vi "Obtain Request Events.vi"(8 "error in (no error)":errorcluster, 10 "Create New?":bool) -> (0 "error out":errorcluster, 2 "UI Manager Request Events":T1)   [LabVIEW 2022 SP3, in "UI Manager.lvlib"]
doc: "This VI Obtains/Creates the Requests events that will be used for other modules to communicate with the module that owns this VI. These Requests events will be accessed only via Public API methods for this module.\n\n<b>NOTE</b>: The contents of this VI are automatically generated and modified by the <b>Tools > Delacor > DQMH</b> utilities. Consider using those utilities instead of making your own modifications to this VI.\n____\nHAMPEL SOFTWARE ENGINEERING v2.6.0 (2023-12-19 10:54)"
uses:
  UI Manager.lvlib
  Request Events--cluster.ctl
  Stop Argument--cluster.ctl
  Show Panel Argument--cluster.ctl
  Hide Panel Argument--cluster.ctl
  Get Module Execution Status Argument--cluster.ctl
  Show Diagram Argument--cluster.ctl
  Set Run-Time Menu Argument--cluster.ctl
  Show HSE-ABOUT Argument--cluster.ctl
  Show PROJECT-ABOUT Argument--cluster.ctl
  Configure Argument--cluster.ctl
  Prepare Argument--cluster.ctl
  Update Status Bar Argument--cluster.ctl
  Trigger System Message Argument--cluster.ctl
  Add Module to Run-Time Menu Argument--cluster.ctl
  Set Modules Argument--cluster.ctl
  Set Modules (Reply Payload)--cluster.ctl
  Register for Module Events Argument--cluster.ctl
  Libraries/hse-libraries/Source/hse-dqmh/Controls/System Message Argument--cluster.ctl
  Libraries/hse-libraries/Source/hse-dqmh/Controls/System Message Source.ctl
  Display another Module UI Argument--cluster.ctl
  Module Display Scenarios.ctl
  Set Run-Time Menu Visibility Argument--cluster.ctl
  Set Window Closeable State Argument--cluster.ctl
  Shutdown Application Argument--cluster.ctl
  Remove Module from Run-Time Menu Argument--cluster.ctl
  Set CLI Arguments Argument--cluster.ctl
  Set CLI Arguments (Reply Payload)--cluster.ctl
  Get CLI Arguments Argument--cluster.ctl
  Get CLI Arguments (Reply Payload)--cluster.ctl
  External Login Argument--cluster.ctl
  Get User Level Argument--cluster.ctl
  Get User Level (Reply Payload)--cluster.ctl
  Libraries/hse-libraries/Source/hse-dqmh/hse-dqmh.lvlib
panel:
  # "NOTE: The contents of this VI are automatically generated and modified by the Tools > Delacor > DQMH utilities. Consider using those utilities instead of making your own modifications to this VI."
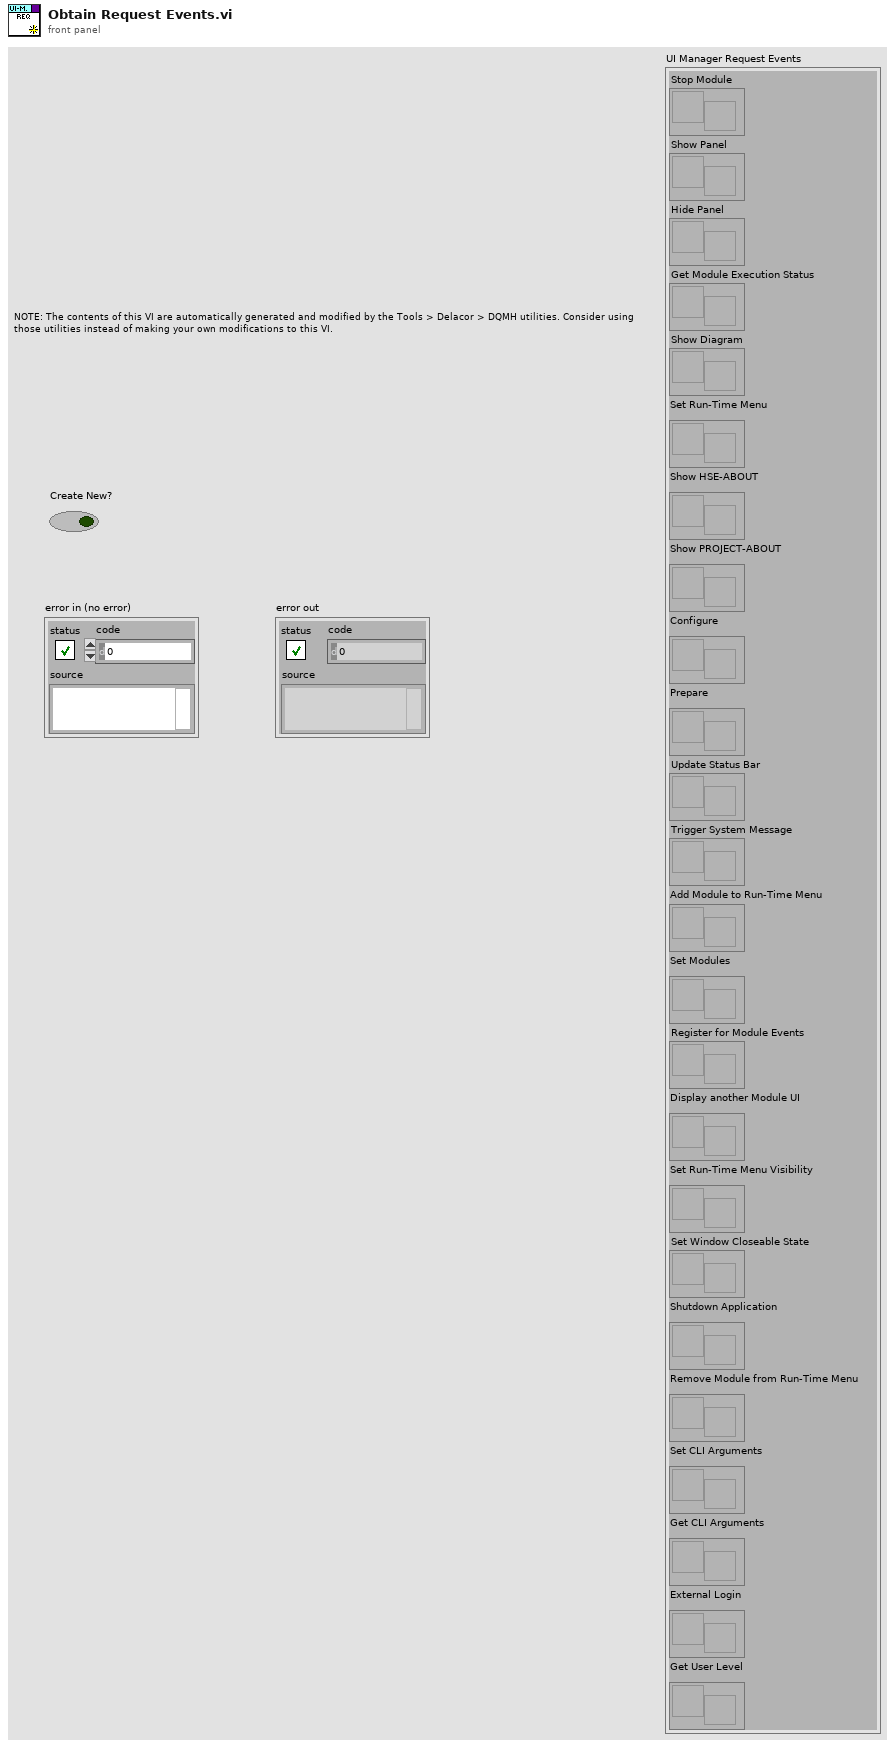
[diagram p1: front panel]
types:
  T1 = typedef "UI Manager.lvlib/Request Events--cluster.ctl" = cluster{"Stop Module":refnum<user-event>, "Show Panel":refnum<user-event>, "Hide Panel":refnum<user-event>, "Get Module Execution Status":refnum<user-event>, "Show Diagram":refnum<user-event>, "Set Run-Time Menu":refnum<user-event>, "Show HSE-ABOUT":refnum<user-event>, "Show PROJECT-ABOUT":refnum<user-event>, "Configure":refnum<user-event>, "Prepare":refnum<user-event>, "Update Status Bar":refnum<user-event>, "Trigger System Message":refnum<user-event>, "Add Module to Run-Time Menu":refnum<user-event>, "Set Modules":refnum<user-event>, "Register for Module Events":refnum<user-event>, "Display another Module UI":refnum<user-event>, "Set Run-Time Menu Visibility":refnum<user-event>, "Set Window Closeable State":refnum<user-event>, "Shutdown Application":refnum<user-event>, "Remove Module from Run-Time Menu":refnum<user-event>, "Set CLI Arguments":refnum<user-event>, "Get CLI Arguments":refnum<user-event>, "External Login":refnum<user-event>, "Get User Level":refnum<user-event>}
  T2 = typedef "UI Manager.lvlib/Get User Level Argument--cluster.ctl" = cluster{"Wait Notifier":refnum<notifier>, "wait for reply":bool}
  T3 = typedef "UI Manager.lvlib/External Login Argument--cluster.ctl" = cluster{"User Name":string, "User Level":string}
  T4 = typedef "UI Manager.lvlib/Get CLI Arguments Argument--cluster.ctl" = cluster{"Wait Notifier":refnum<notifier>, "wait for reply":bool}
  T5 = typedef "UI Manager.lvlib/Set CLI Arguments Argument--cluster.ctl" = cluster{"CLI Arguments":string[], "Wait Notifier":refnum<notifier>, "wait for reply":bool}
  T6 = typedef "UI Manager.lvlib/Remove Module from Run-Time Menu Argument--cluster.ctl" = cluster{"Module DQMH Path":path}
  T7 = typedef "UI Manager.lvlib/Shutdown Application Argument--cluster.ctl" = cluster{"User Confirm?":bool}
  T8 = typedef "UI Manager.lvlib/Set Window Closeable State Argument--cluster.ctl" = cluster{"Closeable?":bool}
  T9 = typedef "UI Manager.lvlib/Set Run-Time Menu Visibility Argument--cluster.ctl" = cluster{"Visible?":bool}
  T10 = typedef "UI Manager.lvlib/Display another Module UI Argument--cluster.ctl" = cluster{"Module DQMH Path":path, "Display Scenario":T11}
  T11 = typedef "UI Manager.lvlib/Module Display Scenarios.ctl" = enum16{"Stand-Alone", "Managed"}
  T12 = typedef "UI Manager.lvlib/Register for Module Events Argument--cluster.ctl" = cluster{"System Messages":refnum<user-event>[]}
  T13 = typedef "UI Manager.lvlib/Set Modules Argument--cluster.ctl" = cluster{"Module Paths":path[], "Wait Notifier":refnum<notifier>, "wait for reply":bool}
  T14 = typedef "UI Manager.lvlib/Add Module to Run-Time Menu Argument--cluster.ctl" = cluster{"Module DQMH Path":path, "Module Descriptor":string}
  T15 = typedef "UI Manager.lvlib/Trigger System Message Argument--cluster.ctl" = cluster{"Boolean":bool}
  T16 = typedef "UI Manager.lvlib/Update Status Bar Argument--cluster.ctl" = cluster{"Status Message":string}
  T17 = typedef "UI Manager.lvlib/Prepare Argument--cluster.ctl" = cluster{"Boolean":bool}
  T18 = typedef "UI Manager.lvlib/Configure Argument--cluster.ctl" = cluster{"Boolean":bool}
  T19 = typedef "UI Manager.lvlib/Show PROJECT-ABOUT Argument--cluster.ctl" = cluster{"Boolean":bool}
  T20 = typedef "UI Manager.lvlib/Show HSE-ABOUT Argument--cluster.ctl" = cluster{"Boolean":bool}
  T21 = typedef "UI Manager.lvlib/Set Run-Time Menu Argument--cluster.ctl" = cluster{"Run-Time Menu Path":path}
  T22 = typedef "UI Manager.lvlib/Hide Panel Argument--cluster.ctl" = cluster{"Hide Panel?":bool}
  T23 = typedef "UI Manager.lvlib/Show Panel Argument--cluster.ctl" = cluster{"Show Panel?":bool}
  T24 = typedef "UI Manager.lvlib/Show Diagram Argument--cluster.ctl" = cluster{"Debug?":bool}
  T25 = typedef "UI Manager.lvlib/Get Module Execution Status Argument--cluster.ctl" = cluster{"Running?":bool}
  T26 = typedef "UI Manager.lvlib/Stop Argument--cluster.ctl" = cluster{"Origin":string, "Exit via Stop Module Req?":bool, "Wait for Module to stop?":bool}
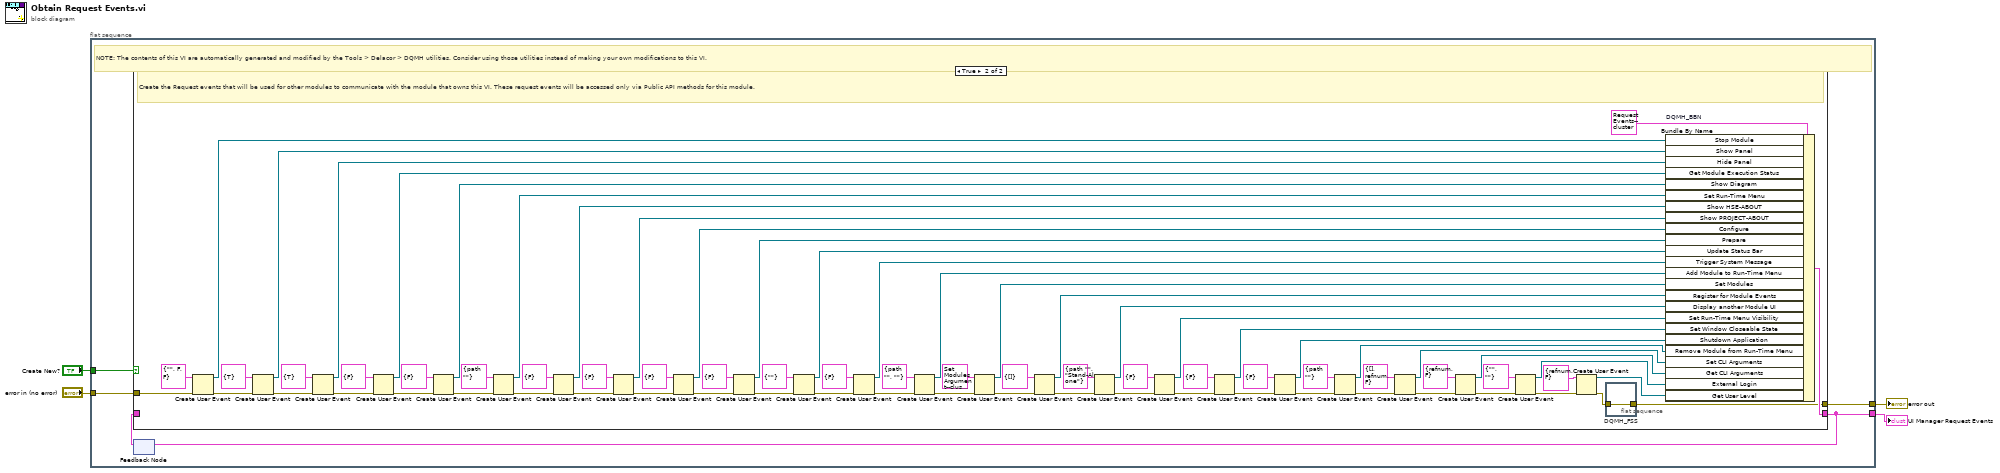
[diagram p0: block diagram]
diagram:
  n1 = flat-sequence {
    tunnel: [w9] -> w4
    tunnel: "error in (no error)" -> [w8]
    tunnel: [w6] -> w2
    tunnel: "Create New?" -> [w5]
    frame #0 {
      # "NOTE: The contents of this VI are automatically generated and modified by the Tools > Delacor > DQMH utilities. Consider using those utilities instead of making your own modifications to this VI."
      n2 = feedback #1() -> (w7:T1)  [unwired: 1 in]
      n3 = case shown="True" w5 {
        tunnel: [w10 w77] -> w9
        tunnel: w8 -> [w10 w87]
        tunnel: [w11 w84] -> w6
        tunnel: w7 -> [w11 _]
        frame False {
          # "Obtain the Request events that were created in a previous call to this VI."
        }
        frame True {
          # "Create the Request events that will be used for other modules to communicate with the module that owns this VI. These request events will be accessed only via Public API methods for this module."
          n4 = Create User Event(user event datatype=T26 {"Origin"="", "Exit via Stop Module Req?"=FALSE, "Wait for Module to stop?"=FALSE} ("Stop Argument"), error in=w87) -> (user event=w85:refnum<user-event>, error out=w82:errorcluster)
          n5 = Create User Event(user event datatype=T23 {"Show Panel?"=TRUE} ("Show Panel Argument"), error in=w82) -> (user event=w81:refnum<user-event>, error out=w80:errorcluster)
          n6 = Create User Event(user event datatype=T22 {"Hide Panel?"=TRUE} ("Hide Panel Argument"), error in=w80) -> (user event=w79:refnum<user-event>, error out=w78:errorcluster)
          n7 = Create User Event(user event datatype=T25 {"Running?"=FALSE} ("Get Module Execution Status Argument"), error in=w78) -> (user event=w75:refnum<user-event>, error out=w76:errorcluster)
          n8 = Create User Event(user event datatype=T24 {"Debug?"=FALSE} ("Show Diagram Argument"), error in=w76) -> (user event=w72:refnum<user-event>, error out=w73:errorcluster)
          n9 = Create User Event(user event datatype=T21 {"Run-Time Menu Path"=path ""} ("Set Run-Time Menu Argument"), error in=w73) -> (user event=w67:refnum<user-event>, error out=w68:errorcluster)
          n10 = Create User Event(user event datatype=T20 {"Boolean"=FALSE} ("Show HSE-ABOUT Argument"), error in=w68) -> (user event=w64:refnum<user-event>, error out=w65:errorcluster)
          n11 = Create User Event(user event datatype=T19 {"Boolean"=FALSE} ("Show PROJECT-ABOUT Argument"), error in=w65) -> (user event=w61:refnum<user-event>, error out=w62:errorcluster)
          n12 = Create User Event(user event datatype=T18 {"Boolean"=FALSE} ("Configure Argument"), error in=w62) -> (user event=w58:refnum<user-event>, error out=w59:errorcluster)
          n13 = Create User Event(user event datatype=T17 {"Boolean"=FALSE} ("Prepare Argument"), error in=w59) -> (user event=w55:refnum<user-event>, error out=w56:errorcluster)
          n14 = Create User Event(user event datatype=T16 {"Status Message"=""} ("Update Status Bar Argument"), error in=w56) -> (user event=w52:refnum<user-event>, error out=w53:errorcluster)
          n15 = Create User Event(user event datatype=T15 {"Boolean"=FALSE} ("Trigger System Message Argument"), error in=w53) -> (user event=w49:refnum<user-event>, error out=w50:errorcluster)
          n16 = Create User Event(user event datatype=T14 {"Module DQMH Path"=path "", "Module Descriptor"=""} ("Add Module to Run-Time Menu Argument"), error in=w50) -> (user event=w46:refnum<user-event>, error out=w47:errorcluster)
          n17 = Create User Event(user event datatype=T13 {"Module Paths"=[path "Modules/Dummie"], "Wait Notifier"=refnum, "wait for reply"=FALSE} ("Set Modules Argument"), error in=w47) -> (user event=w43:refnum<user-event>, error out=w44:errorcluster)
          n18 = Create User Event(user event datatype=T12 {"System Messages"=[]} ("Register for Module Events Argument"), error in=w44) -> (user event=w40:refnum<user-event>, error out=w41:errorcluster)
          n19 = Create User Event(user event datatype=T10 {"Module DQMH Path"=path "", "Display Scenario"=enum."Stand-Alone"} ("Display Module UI Argument"), error in=w41) -> (user event=w37:refnum<user-event>, error out=w38:errorcluster)
          n20 = Create User Event(user event datatype=T9 {"Visible?"=FALSE} ("Set Run-Time Menu Visibility Argument"), error in=w38) -> (user event=w34:refnum<user-event>, error out=w35:errorcluster)
          n21 = Create User Event(user event datatype=T8 {"Closeable?"=FALSE} ("Set Window Closeable State Argument"), error in=w35) -> (user event=w31:refnum<user-event>, error out=w32:errorcluster)
          n22 = Create User Event(user event datatype=T7 {"User Confirm?"=FALSE} ("Shutdown Application Argument"), error in=w32) -> (user event=w28:refnum<user-event>, error out=w29:errorcluster)
          n23 = Create User Event(user event datatype=T6 {"Module DQMH Path"=path ""} ("Remove Module from Run-Time Menu Argument"), error in=w29) -> (user event=w25:refnum<user-event>, error out=w26:errorcluster)
          n24 = Create User Event(user event datatype=T5 {"CLI Arguments"=[], "Wait Notifier"=refnum, "wait for reply"=FALSE} ("Broadcast Arguments Argument"), error in=w26) -> (user event=w22:refnum<user-event>, error out=w23:errorcluster)
          n25 = Create User Event(user event datatype=T4 {"Wait Notifier"=refnum, "wait for reply"=FALSE} ("Get CLI Arguments Argument"), error in=w23) -> (user event=w19:refnum<user-event>, error out=w20:errorcluster)
          n26 = Create User Event(user event datatype=T3 {"User Name"="", "User Level"=""} ("External Login Argument"), error in=w20) -> (user event=w16:refnum<user-event>, error out=w17:errorcluster)
          n27 = Create User Event(user event datatype=T2 {"Wait Notifier"=refnum, "wait for reply"=FALSE} ("Get User Level Argument"), error in=w17) -> (user event=w13:refnum<user-event>, error out=w14:errorcluster)
          n28 = flat-sequence "DQMH_FSS" {
            tunnel: w14 -> [w88]
            tunnel: [w88] -> w77
            frame #0 {
            }
          }
          n29 = Bundle By Name "DQMH_BBN"(cluster=T1 {"Stop Module"=refnum, "Show Panel"=refnum, "Hide Panel"=refnum, "Get Module Execution Status"=refnum, "Show Diagram"=refnum, "Set Run-Time Menu"=refnum, "Show HSE-ABOUT"=refnum, "Show PROJECT-ABOUT"=refnum, "Configure"=refnum, "Prepare"=refnum, "Update Status Bar"=refnum, "Trigger System Message"=refnum, "Add Module to Run-Time Menu"=refnum, "Set Modules"=refnum, "Register for Module Events"=refnum, "Display another Module UI"=refnum, "Set Run-Time Menu Visibility"=refnum, "Set Window Closeable State"=refnum, "Shutdown Application"=refnum, "Remove Module from Run-Time Menu"=refnum, "Set CLI Arguments"=refnum, "Get CLI Arguments"=refnum, "External Login"=refnum, "Get User Level"=refnum} ("output cluster"), "Stop Module"=w85, "Show Panel"=w81, "Hide Panel"=w79, "Get Module Execution Status"=w75, "Show Diagram"=w72, "Set Run-Time Menu"=w67, "Show HSE-ABOUT"=w64, "Show PROJECT-ABOUT"=w61, "Configure"=w58, "Prepare"=w55, "Update Status Bar"=w52, "Trigger System Message"=w49, "Add Module to Run-Time Menu"=w46, "Set Modules"=w43, "Register for Module Events"=w40, "Display another Module UI"=w37, "Set Run-Time Menu Visibility"=w34, "Set Window Closeable State"=w31, "Shutdown Application"=w28, "Remove Module from Run-Time Menu"=w25, "Set CLI Arguments"=w22, "Get CLI Arguments"=w19, "External Login"=w16, "Get User Level"=w13) -> (w84:T1)
        }
      }
      n30 = feedback-in #1(w6) -> ()
    }
  }
  "UI Manager Request Events" <- w2
  "error out" <- w4
